vi "read tcp devs loop.vi"(8 "error in (no error)":errorcluster, 11 "Data in":T3) -> (0 "error out":errorcluster, 3 "Devs connected":string[](array[string]))   [LabVIEW 2020]
uses:
  tcp shot sender queue.ctl
  TCP Multiple Connections State.ctl
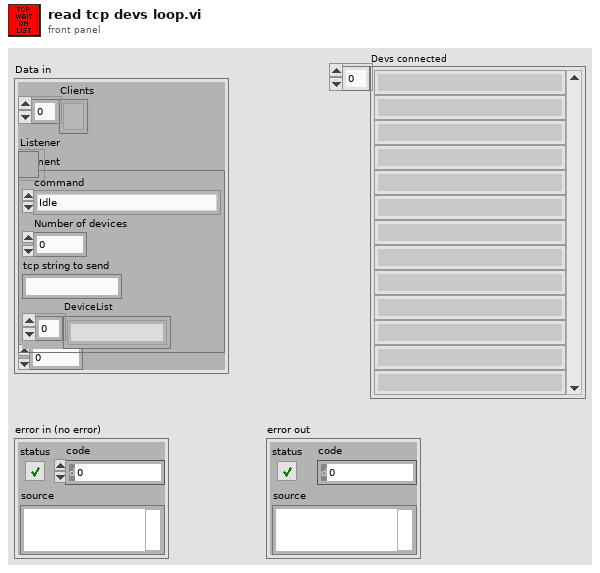
[diagram p1: front panel]
types:
  T1 = typedef "tcp shot sender queue.ctl" = cluster{"command":T2, "Number of devices":i32, "tcp string to send":string, "DeviceList":string[]}
  T2 = typedef "TCP Multiple Connections State.ctl" = enum16{"Idle", "Initialize", "Start Scan", "Send Data", "Stop", "End Scan"}
  T3 = cluster{"Clients":refnum<k5>[], "Listener":refnum<k5>, "element":T1, "startscan tick":u32}
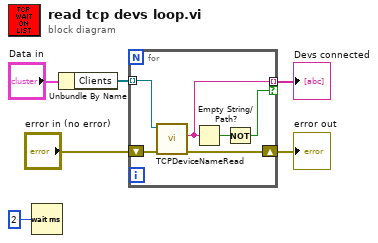
[diagram p0: block diagram]
diagram:
  n1 = Wait (ms)(milliseconds to wait=u32 2) -> ()  [unwired: 1 out]
  n2 = Unbundle By Name("Data in") -> ("Clients"=w2:refnum<k5>[])
  n3 = for {
    tunnel: w2 -> [w11] mode=indexing
    shift-right: [w10] -> w6
    shift-left: "error in (no error)" -> [w12]
    tunnel: [w8] -> w1 mode=indexing if=w7
    n4 = call "TCPDeviceNameRead.vi"("error in (no error)"=w12, "connection ID"=w11) -> ("error out"=w10:errorcluster, "TCPDeviceName"=w8:string)  [unwired: 6 in, 2 out]
    n5 = Empty String/Path?(string/path=w8) -> (empty?=w9:bool)
    n6 = Not(x=w9) -> (.not. x?=w7:bool)
  }
  "error out" <- w6
  "Devs connected" <- w1
